vi "Untitled 3333.vi"() -> ()   [LabVIEW 2015]
uses:
  actors/world/typedefs/worldCell_cluster.ctl
  actors/world/typedefs/markValue_cluster.ctl
  actors/world/typedefs/markValue.ctl
  actors/world/typedefs/markVolume.ctl
  actors/world/typedefs/amountOfFood.ctl
  actors/world/typedefs/anthillType_enum.ctl
  PolyVIEW.lvclass
  actors/world/world.lvlib
panel:
  out "Numeric":dbl
  out "Waveform Graph 3":dbl[][](graph)
  out "Waveform Graph 2":dbl[](graph)
  out "Waveform Graph":dbl[](graph)
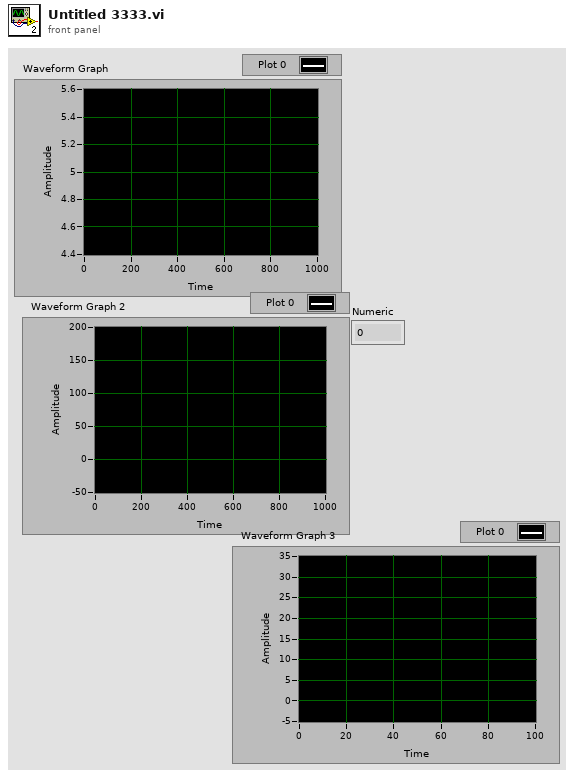
[diagram p1: front panel]
types:
  T1 = typedef "world.lvlib/worldCell_cluster.ctl" = cluster{"marksArray":T2[], "foodAmount":T5, "anthillType":T6, "absoluteHeight":u8}
  T2 = typedef "world.lvlib/markValue_cluster.ctl" = cluster{"value":T3, "volume":T4}
  T3 = typedef "world.lvlib/markValue.ctl" = u8
  T4 = typedef "world.lvlib/markVolume.ctl" = u16
  T5 = typedef "world.lvlib/amountOfFood.ctl" = i32
  T6 = typedef "world.lvlib/anthillType_enum.ctl" = enum16{"empty", "own", "rival"}
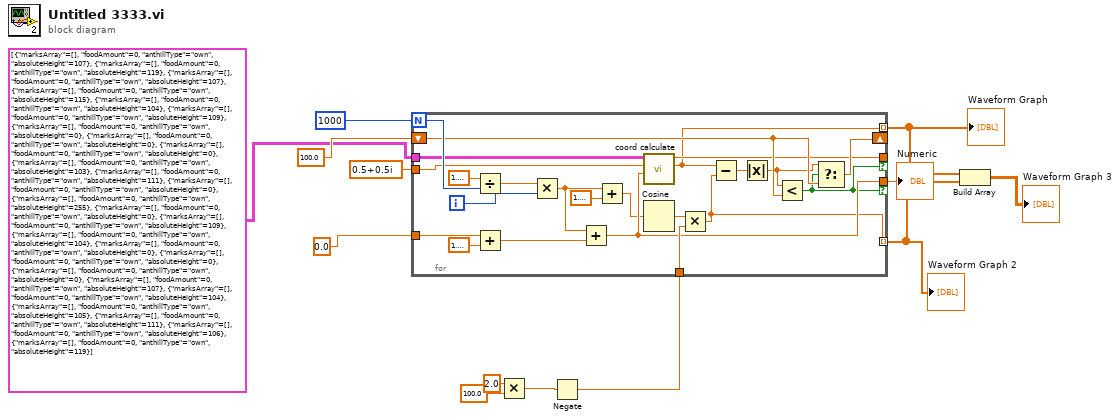
[diagram p0: block diagram]
diagram:
  n1 = Multiply(x=2.0, y=100.0) -> (x*y=w7:dbl)
  n2 = Negate(x=w7) -> (-x=w6:dbl)
  n3 = for {
    N: 1000 -> [w34]
    tunnel: w6 -> [w35]
    tunnel: T1[][] [[{"marksArray"=[], "foodAmount"=0, "anthillType"=enum."own", "absoluteHeight"=107}, {"marksArray"=[], "foodAmount"=0, "anthillType"=enum."own", "absoluteHeight"=119}, {"marksArray"=[], "foodAmount"=0, "anthillType"=enum."own", "absoluteHeight"=107}, {"marksArray"=[], "foodAmount"=0, "anthillType"=enum."own", "absoluteHeight"=115}, {"marksArray"=[], "foodAmount"=0, "anthillType"=enum."own", "absoluteHeight"=104}], [{"marksArray"=[], "foodAmount"=0, "anthillType"=enum."own", "absoluteHeight"=109}, {"marksArray"=[], "foodAmount"=0, "anthillType"=enum."own", "absoluteHeight"=0}, {"marksArray"=[], "foodAmount"=0, "anthillType"=enum."own", "absoluteHeight"=0}, {"marksArray"=[], "foodAmount"=0, "anthillType"=enum."own", "absoluteHeight"=0}, {"marksArray"=[], "foodAmount"=0, "anthillType"=enum."own", "absoluteHeight"=103}], [{"marksArray"=[], "foodAmount"=0, "anthillType"=enum."own", "absoluteHeight"=111}, {"marksArray"=[], "foodAmount"=0, "anthillType"=enum."own", "absoluteHeight"=0}, {"marksArray"=[], "foodAmount"=0, "anthillType"=enum."own", "absoluteHeight"=255}, {"marksArray"=[], "foodAmount"=0, "anthillType"=enum."own", "absoluteHeight"=0}, {"marksArray"=[], "foodAmount"=0, "anthillType"=enum."own", "absoluteHeight"=109}], [{"marksArray"=[], "foodAmount"=0, "anthillType"=enum."own", "absoluteHeight"=104}, {"marksArray"=[], "foodAmount"=0, "anthillType"=enum."own", "absoluteHeight"=0}, {"marksArray"=[], "foodAmount"=0, "anthillType"=enum."own", "absoluteHeight"=0}, {"marksArray"=[], "foodAmount"=0, "anthillType"=enum."own", "absoluteHeight"=0}, {"marksArray"=[], "foodAmount"=0, "anthillType"=enum."own", "absoluteHeight"=107}], [{"marksArray"=[], "foodAmount"=0, "anthillType"=enum."own", "absoluteHeight"=104}, {"marksArray"=[], "foodAmount"=0, "anthillType"=enum."own", "absoluteHeight"=105}, {"marksArray"=[], "foodAmount"=0, "anthillType"=enum."own", "absoluteHeight"=111}, {"marksArray"=[], "foodAmount"=0, "anthillType"=enum."own", "absoluteHeight"=106}, {"marksArray"=[], "foodAmount"=0, "anthillType"=enum."own", "absoluteHeight"=119}]] ("pieceOfWorld") -> [w31]
    shift-right: [w27] -> _
    shift-left: 100.0 -> [w29]
    tunnel: cdb 0.5+0.5i ("coord") -> [w26]
    tunnel: [w25] -> w1 if=w23
    tunnel: [w24] -> _ if=w23
    tunnel: 0.0 ("home az") -> [w21]
    tunnel: [w15] -> w3 mode=indexing
    tunnel: [w14] -> w4 mode=indexing
    i -> [w33]
    n4 = Divide(x=1.5707963267948966, y=w34) -> (x/y=w32:dbl)
    n5 = Add(x=w21, y=1.5707963267948966) -> (x+y=w19:dbl)
    n6 = Multiply(x=w32, y=w33) -> (x*y=w16:dbl)
    n7 = Add(x=w16, y=w19) -> (x+y=w25:dbl)
    n8 = Add(x=w16, y=1.5707963267948966) -> (x+y=w17:dbl)
    n9 = call "coord calculate.vi"("theta"=w25, "coord"=w26, "pieceOfWorld in"=w31) -> ("length"=w14:dbl, "coord out"=w24:cdb)  [unwired: 7 in]
    n10 = Cosine(x=w17) -> (cos(x)=w36:dbl)
    n11 = Multiply(x=w36, y=w35) -> (x*y=w15:dbl)
    n12 = Subtract(x=w14, y=w15) -> (x-y=w30:dbl)
    n13 = Absolute Value(x=w30) -> (abs(x)=w28:dbl)
    n14 = Less?(x=w28, y=w29) -> (x < y?=w23:bool)
    n15 = Select(t=w28, s=w23, f=w29) -> (s? t:f=w27:dbl)
  }
  "Waveform Graph 2" <- w3
  "Waveform Graph" <- w4
  "Numeric" <- w1
  n16 = Build Array(w4, w3) -> (→"Waveform Graph 3":dbl[][])
